vi "TP_FGV_Config.vi"() -> ()   [LabVIEW 2012]
uses:
  <vilib>/xml/NI_XML.lvlib
  <resource>/objmgr/DOMUserDefRef.rc
panel:
  out "error out":errorcluster
  in  "error in":errorcluster
  in  "Enum":T1(ring)=enum."GetValue"
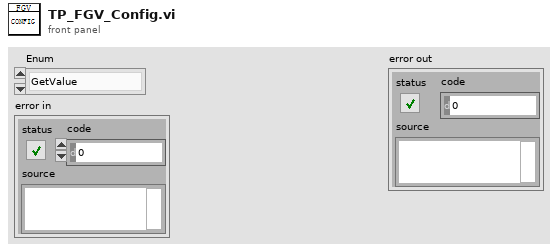
[diagram p1: front panel]
types:
  T1 = enum16{"Init", "GetValue", "SetValue", "Destory"}
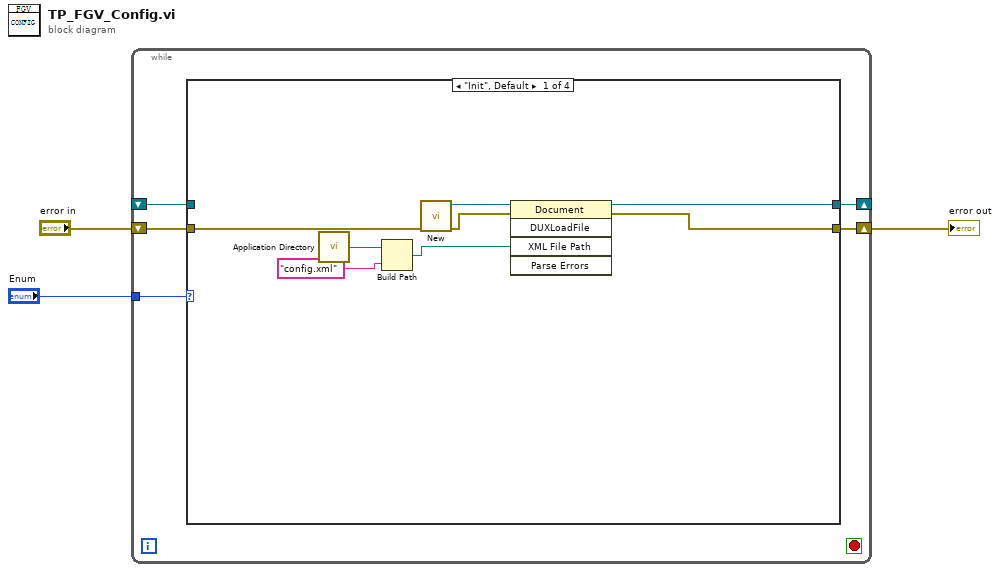
[diagram p0: block diagram]
diagram:
  n1 = while {
    tunnel: "Enum" -> [w8]
    shift-right: [w6] -> _
    shift-left: _ -> [w7]
    shift-right: [w4] -> w1
    shift-left: "error in" -> [w5]
    stop <- _ stop-if-true
    n2 = case shown="\"Init\", Default" w8 {
      tunnel: w7 -> [_ w18 _ _]
      tunnel: [w11 w18 _ _] -> w6
      tunnel: w5 -> [w10 w17 _ _]
      tunnel: [w9 w17 _ _] -> w4
      frame "Init", Default {
        n3 = call <vilib>:"Application Directory.vi"() -> ("Application Directory"=w16:path)
        n4 = Build Path(base path=w16, name or relative path="config.xml") -> (appended path=w13:path)
        n5 = call <vilib>:"New.vi"("error in (no error)"=w10) -> ("error out"=w12:errorcluster, "DOM document out"=w14:refnum<k20>)  [unwired: 7 in]
        n6 = invoke class="Document" method="DUXLoadFile"(reference=w14, error in=w12, "XML File Path"=w13) -> (reference out=w11:refnum<k20>, error out=w9:errorcluster)  [unwired: 2 in, 3 out]
      }
      frame "GetValue" {
      }
      frame "SetValue" {
      }
      frame "Destory" {
      }
    }
  }
  "error out" <- w1
